vi "10-Tap 8-bit Camera with DRAM (FPGA).vi"() -> ()   [LabVIEW 2013]
doc: "This is the FPGA VI for the 10-Tap 8-Bit Camera with DRAM example. This example demonstrates how to acquire images from a 10-tap, 8-bit, extended configuration, Camera Link camera and transfer the images to the host. This example supports area scan and line scan cameras for both continuous and finite acquisitions.\n\nThis example also demonstrates the use of DRAM as a frame buffer for very high speed acquisitions. Data packing and flow-control are also employed to maximize use of the available DRAM and FIFOs in terms of both memory space and performance.\n\nAdditionally, the example demonstrates the serial server, which allows third-party camera configuration utilities to communicate with the camera using the Camera Link serial interface while this VI is running."
uses:
  <vilib>/rvi/DataTransferAndStorage/Container/XNode/niFpgaContainer.xnode
  <vilib>/Platform/TimedLoop/XDataNode/XDataNode.xnode
  <vilib>/Platform/TimedLoop/XDataNode/timing_clust.ctl
  <vilib>/Platform/TimedLoop/XDataNode/XDNodeRunTimeDep.lvlib
  <vilib>/Platform/TimedLoop/XDataNode/wakeup.ctl
  <vilib>/Platform/TimedLoop/XDataNode/nitl_modes.ctl
  <vilib>/eio/EIONode/EIONode.xnode
  <vilib>/rvi/eio/common/nirviEmuTemplateMethod_errors.vi
  <vilib>/rvi/FIFO/Fifo_Resource/nirvififoEmulationGetNumberOfElementsToRead.vi
  <vilib>/rvi/interface/RandomDataEmulation/nirviRandomDataFpgaReadWriteTemplate.vi
  <vilib>/rvi/FIFO/Fifo_Resource/nirvififoEmulationRead.vi
  <vilib>/rvi/FIFO/Fifo_Resource/nirvififoEmulationWrite.vi
  Common/CL Data to Pixels/10 Tap 8-Bit.vi
  FPGA/10-Tap Data/10-Tap Conversion Enum.ctl
  FPGA/Globals/Accumulated Sector Intensity.vi
  FPGA/Globals/Pixel Location Global.vi
  FPGA/Globals/Sector Parameter Global.vi
  <vilib>/rvi/FIFO/Fifo_Resource/nirvififoEmulationGetNumberOfElementsToWrite.vi
  Common/CL Signal Mapping.ctl
  Common/CL Configuration.ctl
  FPGA/Sector/Accumulate/Sector Parameter Cluster.ctl
panel:
  in  "Right End Angle Duty Cycle":fxp<+,8,0>
  in  "Right Start Angle Duty Cycle":fxp<+,8,0>
  in  "Left End Angle Duty Cycle":fxp<+,8,0>
  in  "Left Start Angle Duty Cycle":fxp<+,8,0>
  in  "X Resolution":u16=1000
  in  "Y Resolution":u16=1000
  out "Analysis Ticks":u32
  out "Right Sector Edge":u8
  out "Left Sector Edge":u8
  in  "[Average BG Intensity]":u8[](array[numeric])=[0, 0, 0, 0, 0, 0, 0, 0, 0, 0, 0, 0, 0, 0, 0, 0, 0, 0, 0, 0, 0, 0, 0, 0, 0, 0, 0, 0, 0, 0, 0, 0]
  in  "Sector Threshold":u8
  in  "# of Frames to Average":u8
  in  "Sector Parameters Right":T1={"Start Angle"=0.0, "End Angle"=0.4708251953125, "Inner Radius"=309, "Outter Radius"=405, "Hinge X"=685, "Hinge Y"=527, "NumWingSectors"=8}
  in  "Sector Parameters Left":T1={"Start Angle"=0.65740966796875, "End Angle"=0.99468994140625, "Inner Radius"=309, "Outter Radius"=405, "Hinge X"=464, "Hinge Y"=534, "NumWingSectors"=8}
  in  "CL Config.Configuration":T2=enum."Full"
  in  "CL Config.Signal Mapping":T3=enum."Basler 10-tap"
  in  "CL Config.Line Scan":bool
  in  "CL Config.DVAL Active High":bool=TRUE
  in  "CL Config.LVAL Active High":bool=TRUE
  in  "CL Config.FVAL Active High":bool=TRUE
  in  "CL Config.Spare Active High":bool=TRUE
  in  "Acq Control.Line Scan Height":u32
  in  "Acq Control.Frames To Acq":u32
  in  "Acq Control.Acquire":bool
  in  "Acq Control.Cancel Acq":bool
  in  "Acq Control.Ignore DVAL":bool
  in  "Acq Control.Initialize":bool
  out "Acq Status.Acq In Progress":bool
  out "Acq Status.Clocks Per Line":u32
  out "Acq Status.Frames Acq'd":u32
  out "Acq Status.Lines Per Frame":u32
  out "Acq Status.DMA Write Timeout":bool
  out "Acq Status.Initialized":bool
  in  "UART.Baud Rate":u8
  in  "UART.Transmit":bool
  in  "UART.Tx Data":u8[](array[numeric])=[0, 0, 0, 0, 0, 0, 0, 0, 0, 0] format="%02x"
  in  "UART.Set Baud Rate":bool
  in  "UART.Byte Mode":bool=TRUE
  out "UART.Rx Ready":bool
  out "UART.Break Indicator":bool
  out "UART.Framing Error":bool
  out "UART.Overrun Error":bool
  out "UART.Tx Ready":bool
  out "UART.Rx Data":u8 format="%02x"
  in  "UART.Receive":bool
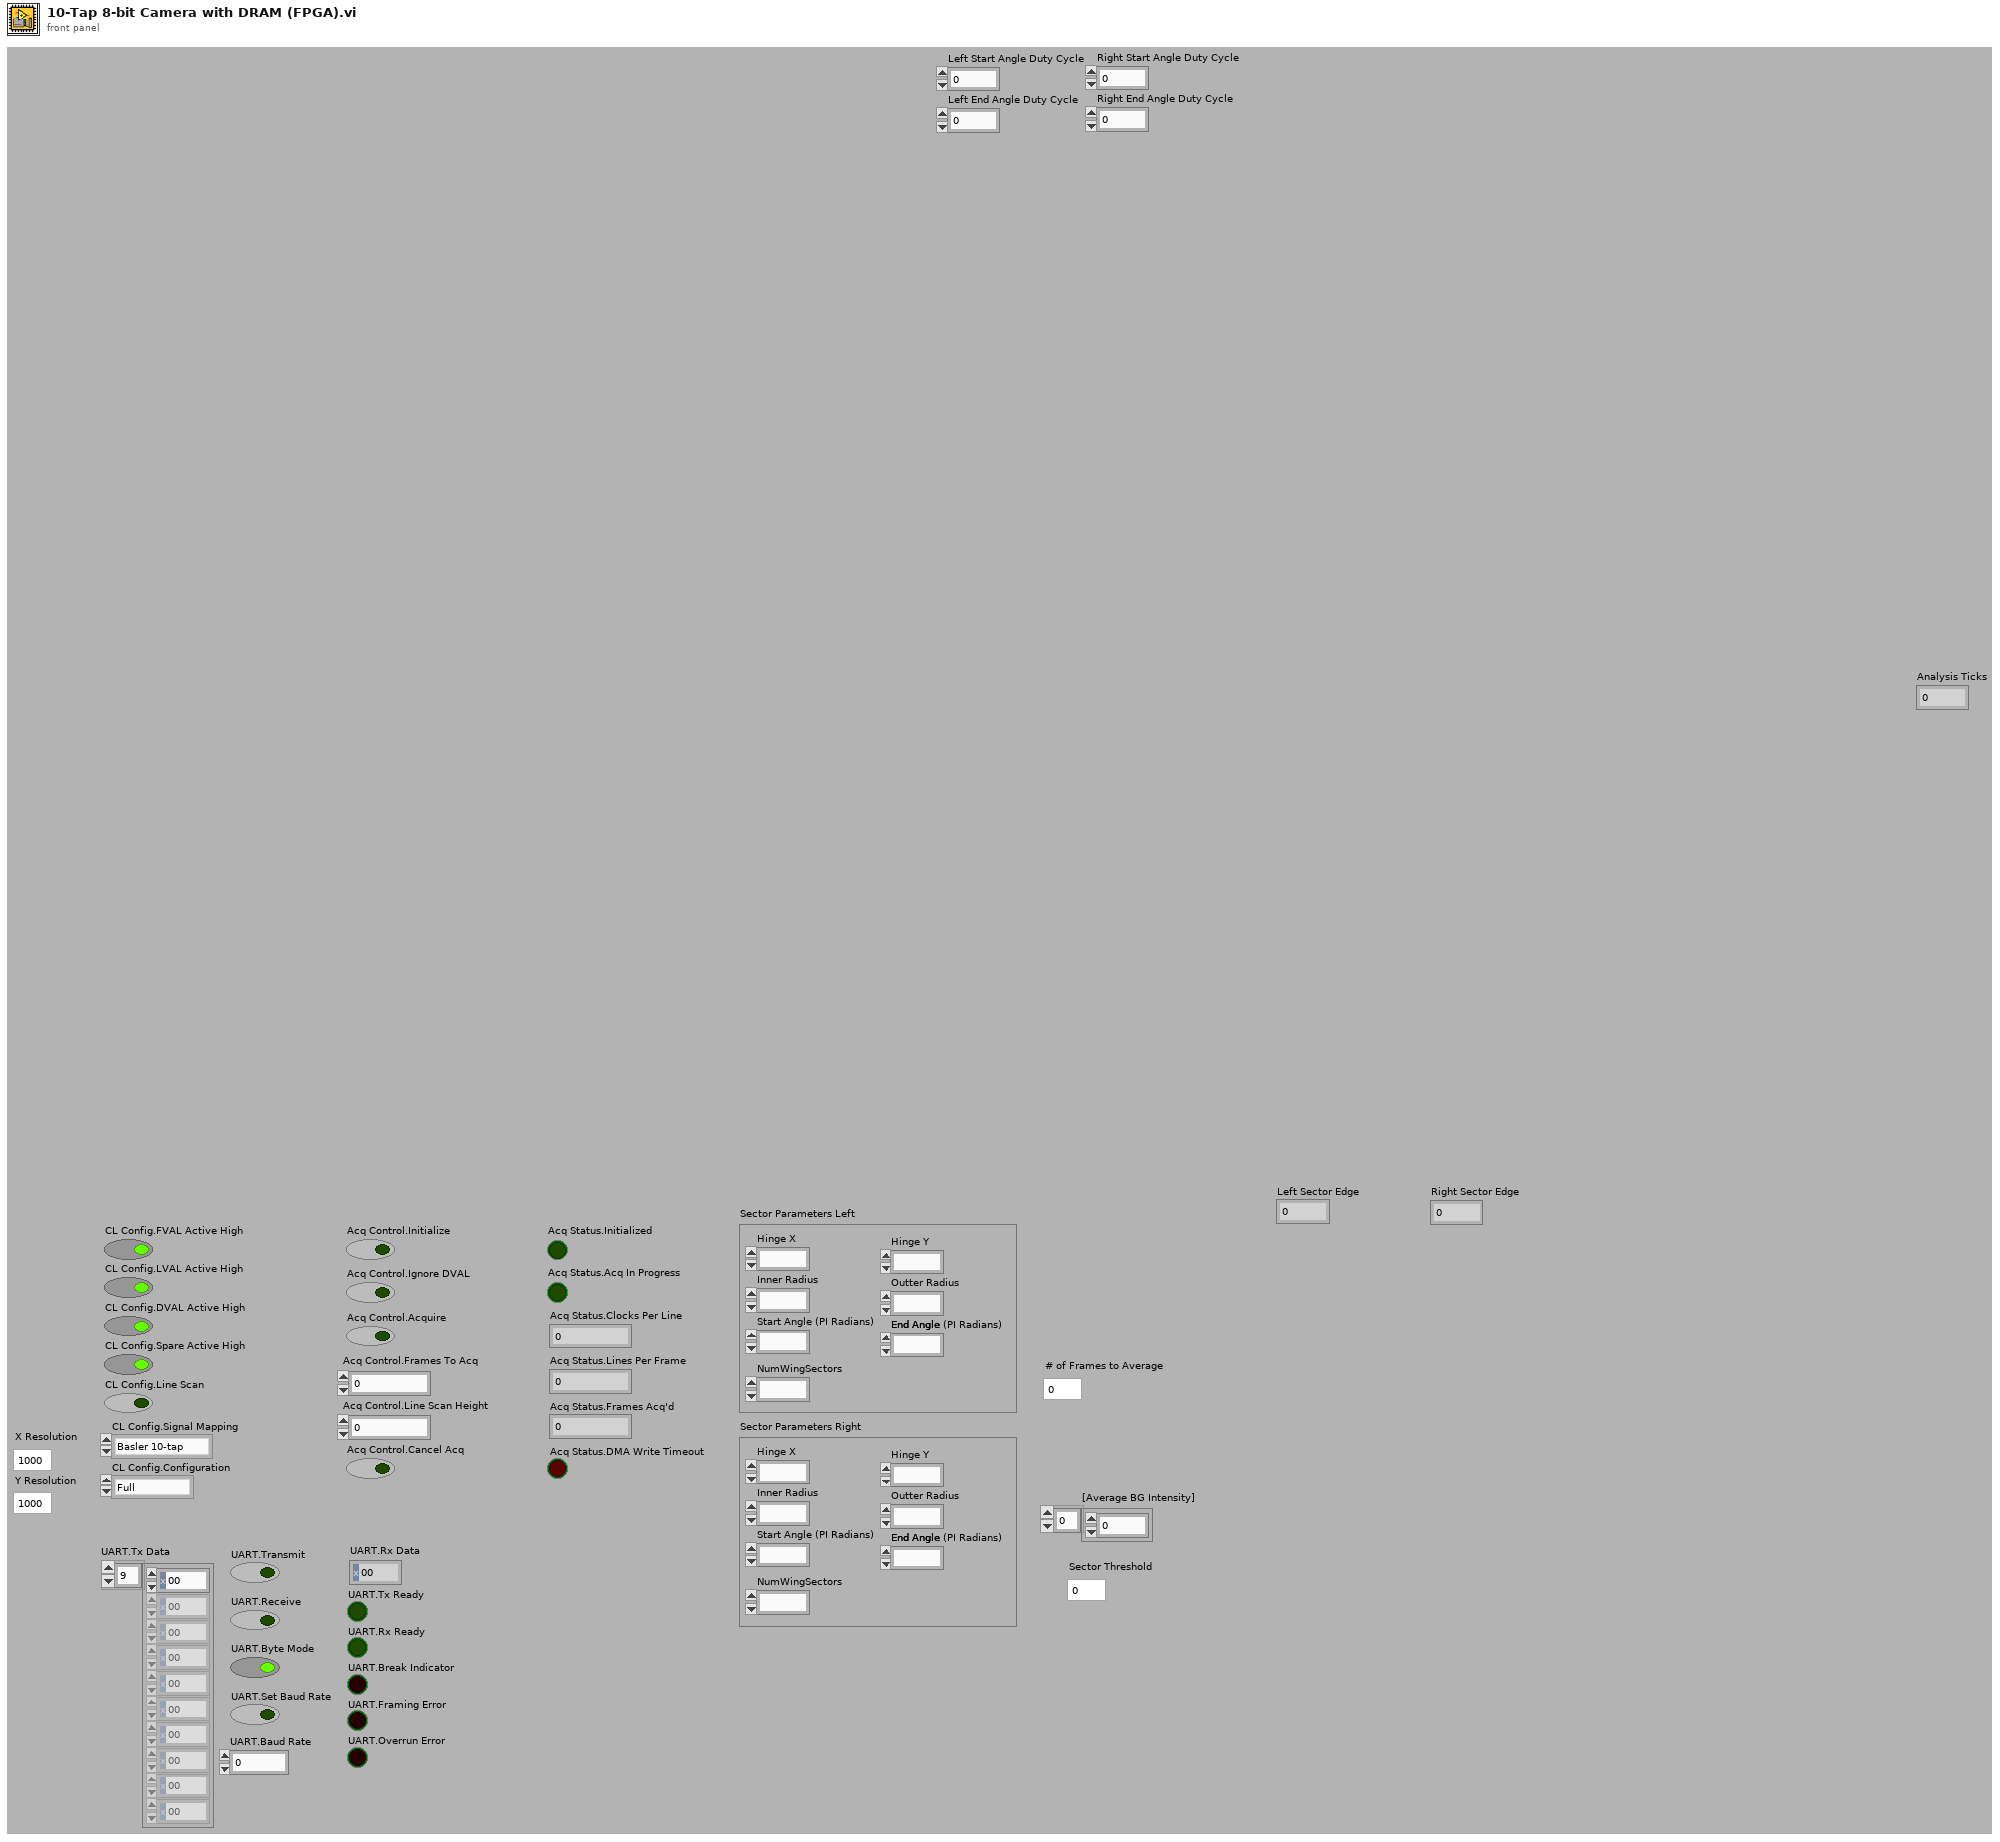
[diagram p1: front panel]
types:
  T1 = typedef "Sector Parameter Cluster.ctl" = cluster{"Start Angle":fxp<+/-,17,2>, "End Angle":fxp<+,17,3>, "Inner Radius":u16, "Outter Radius":u16, "Hinge X":u16, "Hinge Y":u16, "NumWingSectors":u8}
  T2 = typedef "CL Configuration.ctl" = enum8{"Base", "Medium", "Full"}
  T3 = typedef "CL Signal Mapping.ctl" = enum8{"Standard", "Basler 10-tap", "Vosskühler 10-tap"}
  T4 = typedef "XDNodeRunTimeDep.lvlib/timing_clust.ctl" = cluster{"Expected End [f-1]":u64, "Actual End [f-1]":u64, "Finished Late? [f-1]":bool, "Expected End [i-1]":u64, "Actual End [i-1]":u64, "Finished Late? [i-1]":bool, "Expected Start [i]":u64, "Actual Start [i]":u64, "Expected Start [f]":u64, "Actual Start [f]":u64, "Source Name":string, "Structure Name":string, "Period":i64, "Deadline":i64, "Offset":i64, "Start":i64, "Priority":i32, "Timeout":i32, "Mode":T5, "Wakeup Reason":T6, "Error":errorcluster, "Source Type":string, "Secondary Source Type":string, "Global End Time":u64, "Global Start Time":u64, "Frame Duration":u64, "Iteration Duration":u64, "Assigned CPU":i32, "I/O Scan Engine Mode":u32}
  T5 = typedef "XDNodeRunTimeDep.lvlib/nitl_modes.ctl" = enum32{"No Change", "Process missed periods, maintain original phase", "Discard missed periods, maintain original phase", "Process missed periods, ignore original phase", "Discard missed periods, ignore original phase"}
  T6 = typedef "XDNodeRunTimeDep.lvlib/wakeup.ctl" = enum32{"Normal", "Aborted", "Asynchronous wakeup", "Timing source error", "Timed loop error", "Timeout"}
  T7 = typedef "10-Tap Conversion Enum.ctl" = enum16{"10-Tap to 16 and 64", "16 and 64 to 10-Tap"}
  T8 = cluster{"Enables Valid":bool, "Frame Valid":bool, "Line Valid":bool, "Data Valid":bool}
  T9 = typedef "10-Tap 8-bit Cluster.ctl" = cluster{"Pixel 0":u8, "Pixel 1":u8, "Pixel 2":u8, "Pixel 3":u8, "Pixel 4":u8, "Pixel 5":u8, "Pixel 6":u8, "Pixel 7":u8, "Pixel 8":u8, "Pixel 9":u8}
  T10 = cluster{"Tx Data":u8[], "Transmit":bool, "Receive":bool, "Byte Mode":bool, "Set Baud Rate":bool, "Baud Rate":u8}
  T11 = cluster{"Rx Data":u8, "Turn Off Transmit":bool, "Turn Off Receive":bool, "Turn Off Set Baud Rate":bool, "Tx Ready":bool, "Rx Ready":bool, "Break Indicator":bool, "Framing Error":bool, "Overrun Error":bool}
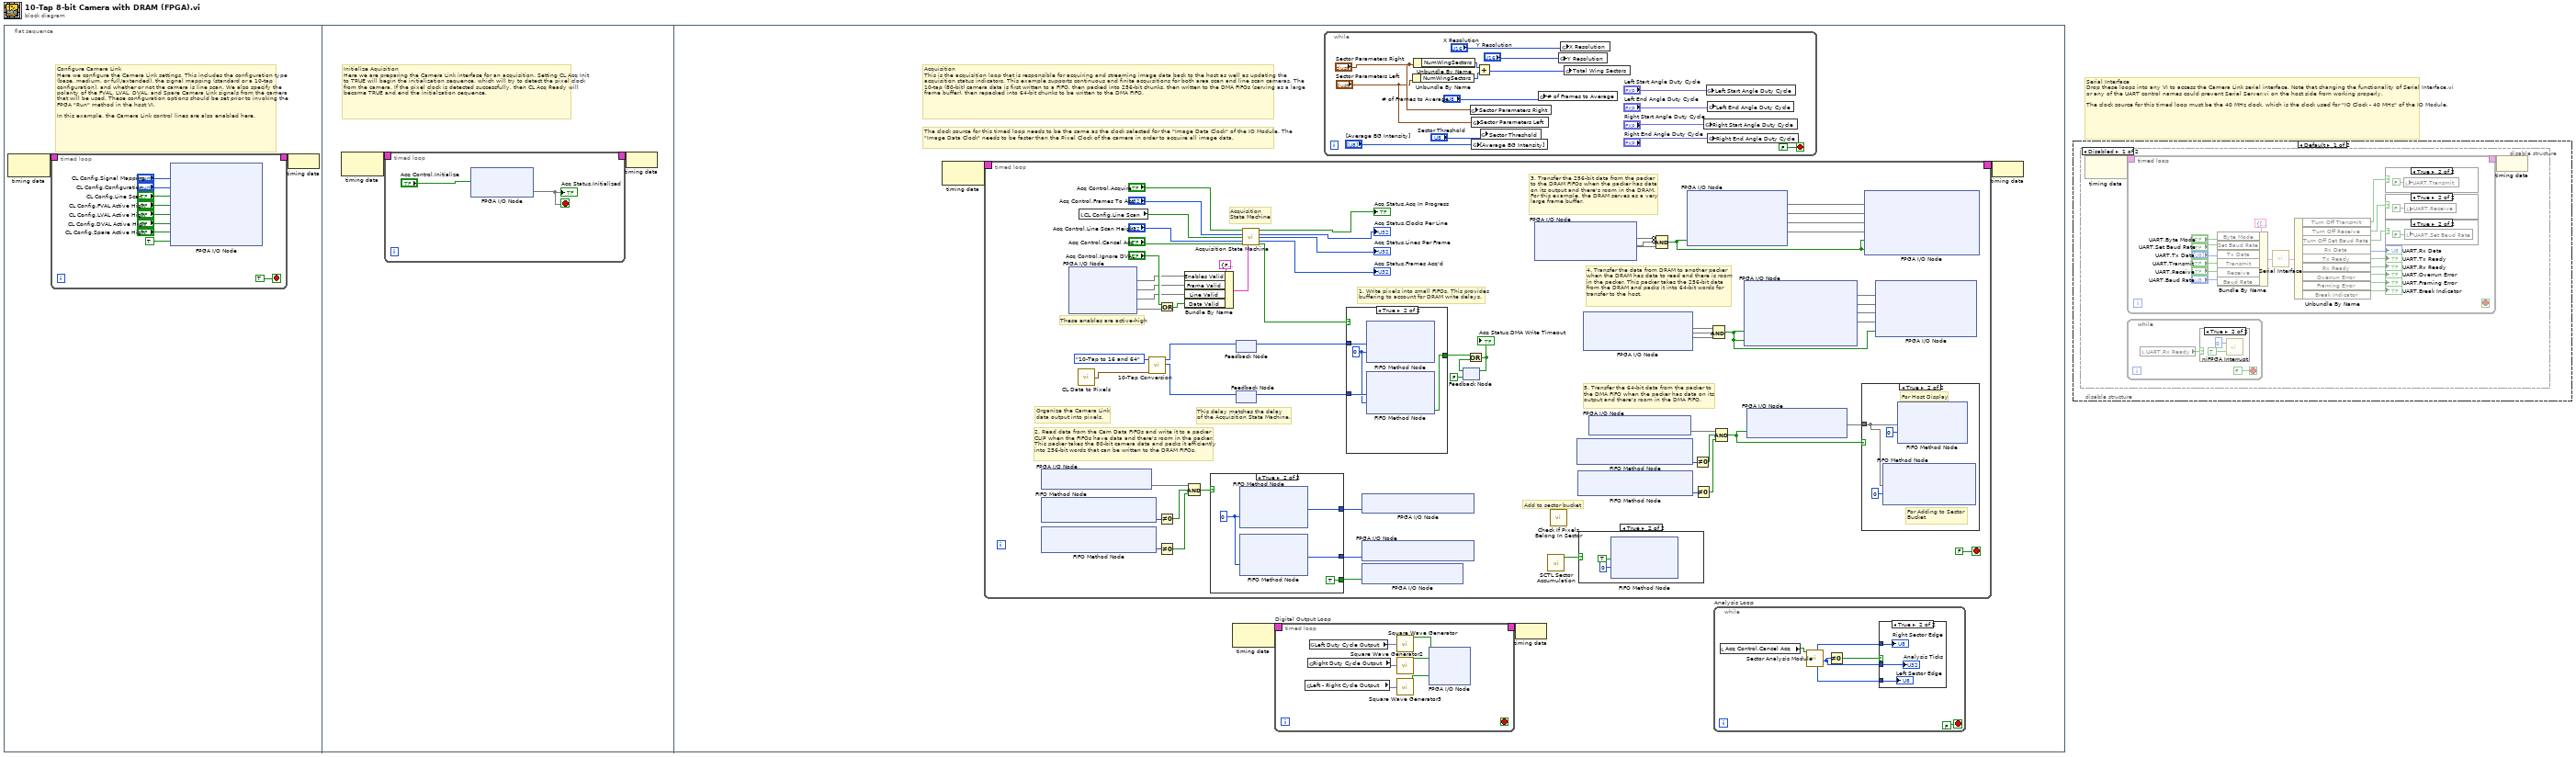
[diagram p0: block diagram]
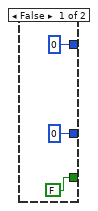
[diagram p11: hidden frame]
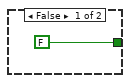
[diagram p12: hidden frame]
diagram:
  # "Serial Interface\nDrop these loops into any VI to access the Camera Link serial interface. Note that changing the functionality of Serial Interface.vi or any of the UART control names could prevent Serial Server.vi on the host side from working properly.\n\nThe clock source for this timed loop must be the 40 MHz clock, which is the clock used for \"IO Clock - 40 MHz\" of the IO Module."
  n1 = flat-sequence {
    frame #0 {
      # "Configure Camera Link\nHere we configure the Camera Link settings. This includes the configuration type (base, medium, or full/extended), the signal mapping (standard or a 10-tap configuration), and whether or not the camera is line scan. We also specify the polarity of the FVAL, LVAL, DVAL, and Spare Camera Link signals from the camera that will be used. These configuration options should be set prior to invoking the FPGA \"Run\" method in the host VI.\n\nIn this example, the Camera Link control lines are also enabled here."
      n2 = node-c288() -> (w2:T4)  [unwired: 1 in]
      n3 = timed-loop {
        timing: w2 -> [_]
        timing-out: [_] -> w1
        stop <- TRUE stop-if-true
        n4 = xnode "FPGA I/O Node"("CL Set Signal Mapping"="CL Config.Signal Mapping", "CL Set Configuration"="CL Config.Configuration", "CL Set Line Scan"="CL Config.Line Scan", "CL Set FVAL Active High"="CL Config.FVAL Active High", "CL Set LVAL Active High"="CL Config.LVAL Active High", "CL Set DVAL Active High"="CL Config.DVAL Active High", "CL Set Spare Active High"="CL Config.Spare Active High", "CL Control Enable"=TRUE ("IO Module\\CL Control Enable")) -> ()  [unwired: 8 in, 8 out]
      }
      n5 = node-c288(w1) -> ()
    }
    frame #1 {
      # "Initialize Aquisition\nHere we are preparing the Camera Link interface for an acquisition. Setting CL Acq Init to TRUE will begin the initialization sequence, which will try to detect the pixel clock from the camera. If the pixel clock is detected successfully, then CL Acq Ready will become TRUE and end the initialzation sequence."
      n6 = node-c288() -> (w17:T4)  [unwired: 1 out]
      n7 = timed-loop {
        timing: w17 -> [_]
        timing-out: [_] -> w16
        stop <- w18 stop-if-true
        n8 = xnode "FPGA I/O Node"("CL Acq Init"="Acq Control.Initialize") -> ("CL Acq Ready"=w18)  [unwired: 2 in, 2 out]
        "Acq Status.Initialized" <- w18
      }
      n9 = node-c288(w16) -> ()
    }
    frame #2 {
      # "The clock source for this timed loop needs to be the same as the clock selected for the \"Image Data Clock\" of the IO Module. The \"Image Data Clock\" needs to be faster than the Pixel Clock of the camera in order to acquire all image data."
      # "Acquisition\nThis is the acquisition loop that is responsible for acquiring and streaming image data back to the host as well as updating the acquisition status indicators. This example supports continuous and finite acquisitions for both area scan and line scan cameras. The 10-tap (80-bit) camera data is first written to a FIFO, then packed into 256-bit chunks, then written to the DMA FIFOs (serving as a large frame buffer), then repacked into 64-bit chunks to be written to the DMA FIFO."
      n10 = node-c288() -> (w27:T4)  [unwired: 1 in]
      n11 = timed-loop {
        timing: w27 -> [_]
        timing-out: [_] -> w26
        stop <- FALSE stop-if-true
        # "These enables are active-high"
        # "Acquisition\nState Machine"
        # "2. Read data from the Cam Data FIFOs and write it to a packer\nCLIP when the FIFOs have data and there's room in the packer.\nThis packer takes the 80-bit camera data and packs it efficiently\ninto 256-bit words that can be written to the DRAM FIFOs."
        # "Organize the Camera Link\ndata output into pixels."
        # "This delay matches the delay\nof the Acquisition State Machine."
        # "Add to sector bucket"
        # "5. Transfer the 64-bit data from the packer to\nthe DMA FIFO when the packer has data on its\noutput and there's room in the DMA FIFO."
        # "4. Transfer the data from DRAM to another packer\nwhen the DRAM has data to read and there is room\nin the packer. This packer takes the 256-bit data\nfrom the DRAM and packs it into 64-bit words for\ntransfer to the host."
        # "3. Transfer the 256-bit data from the packer\nto the DRAM FIFOs when the packer has data\non its output and there's room in the DRAM.\nFor this example, the DRAM serves as a very\nlarge frame buffer."
        # "1. Write pixels into small FIFOs. This provides\nbuffering to account for DRAM write delays."
        n12 = xnode "FPGA I/O Node"() -> ("Pack 80 to 256\\Ready For Write"=w96)  [unwired: 1 in, 1 out]
        n13 = xnode ("FIFO Method Node")() -> ("Number of Elements to Read"=w100:u32)  [unwired: 1 in, 1 out]
        n14 = xnode ("FIFO Method Node")() -> ("Number of Elements to Read"=w99:u32)  [unwired: 1 in, 1 out]
        n15 = xnode "FPGA I/O Node"() -> ("CL Output Valid"=w54, "CL Frame Valid"=w55, "CL Line Valid"=w56, "CL Data Valid"=w59)  [unwired: 4 in, 4 out]
        n16 = call-poly "CL Data to Pixels.vi"() -> ("Pixels"=w47:T9)  [unwired: 1 in]
        n17 = local read "CL Config.Line Scan"() -> (w62:bool)
        n18 = call "10-Tap Conversion.vi"("10 Tap In"=w47, "Operation"=10-Tap_Conversion_Enum."10-Tap to 16 and 64") -> ("64 Bit Out"=w48:u64, "16 Bit Out"=w49:u16)  [unwired: 7 in, 1 out]
        n19 = Or(x="Acq Control.Ignore DVAL", y=w59) -> (x .or. y?=w60:bool)
        n20 = Not Equal To 0?(x=w100) -> (x != 0?=w94:bool)
        n21 = Not Equal To 0?(x=w99) -> (x != 0?=w93:bool)
        n22 = Bundle By Name(cluster=T8 {"Enables Valid"=FALSE, "Frame Valid"=FALSE, "Line Valid"=FALSE, "Data Valid"=FALSE} ("Enables"), "Enables Valid"=w54, "Frame Valid"=w55, "Line Valid"=w56, "Data Valid"=w60) -> (w57:T8)
        n23 = Compound Arithmetic op=AND(w96, w94, w93) -> (w95:bool)
        n24 = case shown="True" w95 {
          tunnel: [u16 0 ("Element") w119] -> w101
          tunnel: [u64 0 ("Element") w118] -> w97
          tunnel: [FALSE TRUE] -> w98
          frame False {
          }
          frame True {
            w117 = 0 ("Timeout")
            n25 = xnode ("FIFO Method Node")("Timeout"=w117) -> ("Element"=w119:u16)  [unwired: 1 in, 2 out]
            n26 = xnode ("FIFO Method Node")("Timeout"=w117) -> ("Element"=w118:u64)  [unwired: 1 in, 2 out]
          }
        }
        n27 = feedback #1() -> (w102:u16)  [unwired: 1 in]
        n28 = feedback-in #1(w49) -> ()
        n29 = feedback #2() -> (w107:u64)  [unwired: 1 in]
        n30 = feedback-in #2(w48) -> ()
        n31 = call "Acquisition State Machine.vi"("Acquire"="Acq Control.Acquire", "Frames to Acquire"="Acq Control.Frames To Acq", "Line Scan"=w62, "Line Scan Height"="Acq Control.Line Scan Height", "Cancel Acq"="Acq Control.Cancel Acq", "Enables"=w57) -> ("Acq In Progress"=→"Acq Status.Acq In Progress":bool, "Num Clocks Per Line"=→"Acq Status.Clocks Per Line":u32, "Num Lines Per Frame"=→"Acq Status.Lines Per Frame":u32, "Num Frames Acq'd"=→"Acq Status.Frames Acq'd":u32, "Capture Cycle"=w91:bool)  [unwired: 4 in, 1 out]
        n32 = case shown="True" w91 {
          tunnel: [FALSE ("Timed Out?") w123] -> w105
          tunnel: w107 -> [_ w124]
          tunnel: w102 -> [_ w122]
          frame False {
          }
          frame True {
            w121 = 0 ("Timeout")
            n33 = xnode ("FIFO Method Node")("Element"=w122, "Timeout"=w121) -> ()  [unwired: 1 in, 2 out]
            n34 = xnode ("FIFO Method Node")("Element"=w124, "Timeout"=w121) -> ("Timed Out?"=w123:bool)  [unwired: 1 in, 1 out]
          }
        }
        n35 = xnode "FPGA I/O Node"("Pack 80 to 256\\Data In Upper 16"=w101) -> ()  [unwired: 1 in, 1 out]
        n36 = xnode "FPGA I/O Node"("Pack 80 to 256\\Data In Lower 64"=w97) -> ()  [unwired: 1 in, 1 out]
        n37 = xnode "FPGA I/O Node"("Pack 80 to 256\\Write Enable"=w98) -> ()  [unwired: 1 in, 1 out]
        n38 = feedback #3(FALSE) -> (w104:bool)
        n39 = Or(x=w105, y=w104) -> (x .or. y?=w103:bool)
        "Acq Status.DMA Write Timeout" <- w103
        n40 = feedback-in #3(w103) -> ()
        n41 = xnode "FPGA I/O Node"() -> ("DRAM Bank 0\\Full"=w67, "Pack 80 to 256\\Output Valid"=w86)  [unwired: 3 in, 4 out]
        n42 = call "SCTL Sector Accumulation.vi"() -> ("New Data?"=w64:bool)  [unwired: 11 in]
        n43 = call "Check If Pixels Belong In Sector.vi"() -> ()  [unwired: 11 in, 1 out]
        n44 = xnode ("FIFO Method Node")() -> ("Number of Elements to Write"=w69:u32)  [unwired: 1 in, 1 out]
        n45 = xnode ("FIFO Method Node")() -> ("Number of Elements to Write"=w66:u32)  [unwired: 1 in, 1 out]
        n46 = case shown="True" w64 {
          frame False {
          }
          frame True {
            n47 = xnode ("FIFO Method Node")("Element"=TRUE, "Timeout"=0) -> ()  [unwired: 1 in, 2 out]
          }
        }
        n48 = xnode "FPGA I/O Node"() -> ("DRAM Bank 1\\Data_Available"=w80, "DRAM Bank 0\\Data_Available"=w78, "Pack 256 to 64\\Ready for Write"=w79)  [unwired: 3 in, 3 out]
        n49 = xnode "FPGA I/O Node"() -> ("Pack 256 to 64\\Output Valid"=w71)  [unwired: 1 in, 1 out]
        n50 = Compound Arithmetic op=AND(invert w67, invert w67, w86) -> (w81:bool)
        n51 = xnode "FPGA I/O Node"("Pack 80 to 256\\Read Enable"=w81) -> ("Pack 80 to 256\\Data Out 3"=w85, "Pack 80 to 256\\Data Out 2"=w84, "Pack 80 to 256\\Data Out 1"=w83, "Pack 80 to 256\\Data Out 0"=w82)  [unwired: 5 in, 5 out]
        n52 = Not Equal To 0?(x=w69) -> (x != 0?=w70:bool)
        n53 = Not Equal To 0?(x=w66) -> (x != 0?=w65:bool)
        n54 = Compound Arithmetic op=AND(w80, w78, w79) -> (w73:bool)
        n55 = Compound Arithmetic op=AND(w71, w70, w65) -> (w68:bool)
        n56 = xnode "FPGA I/O Node"("DRAM Bank 1\\Read"=w73, "DRAM Bank 0\\Read"=w73) -> ("DRAM Bank 1\\Read_Data_Upper"=w77, "DRAM Bank 1\\Read_Data_Lower"=w76, "DRAM Bank 0\\Read_Data_Upper"=w75, "DRAM Bank 0\\Read_Data_Lower"=w74)  [unwired: 6 in, 6 out]
        n57 = xnode "FPGA I/O Node"("Pack 256 to 64\\Read Enable"=w68) -> ("Pack 256 to 64\\Data Out 64"=w72)  [unwired: 2 in, 2 out]
        n58 = case shown="True" w68 {
          tunnel: w72 -> [_ w111]
          frame False {
          }
          frame True {
            # "For Adding to Sector \nBucket"
            # "For Host Display"
            n59 = xnode ("FIFO Method Node")("Element"=w111, "Timeout"=0) -> ()  [unwired: 1 in, 2 out]
            n60 = xnode ("FIFO Method Node")("Element"=w111, "Timeout"=0) -> ()  [unwired: 1 in, 2 out]
          }
        }
        n61 = xnode "FPGA I/O Node"("DRAM Bank 1\\Write_Data_Upper"=w85, "DRAM Bank 1\\Write_Data_Lower"=w84, "DRAM Bank 0\\Write_Data_Upper"=w83, "DRAM Bank 0\\Write_Data_Lower"=w82, "DRAM Bank 1\\Write"=w81, "DRAM Bank 0\\Write"=w81) -> ()  [unwired: 6 in, 6 out]
        n62 = xnode "FPGA I/O Node"("Pack 256 to 64\\Data In 3"=w77, "Pack 256 to 64\\Data In 2"=w76, "Pack 256 to 64\\Data In 1"=w75, "Pack 256 to 64\\Data In 0"=w74, "Pack 256 to 64\\Write Enable"=w73) -> ()  [unwired: 5 in, 5 out]
      }
      n63 = node-c288() -> (w25:T4)  [unwired: 1 in]
      n64 = timed-loop "Digital Output Loop" {
        timing: w25 -> [_]
        timing-out: [_] -> w24
        stop <- _ stop-if-true
        n65 = global read "Sector Parameter Global.vi" "Left - Right Cycle Output"() -> (w40:fxp<+,8,0>)
        n66 = global read "Sector Parameter Global.vi" "Right Duty Cycle Output"() -> (w41:fxp<+,8,0>)
        n67 = global read "Sector Parameter Global.vi" "Left Duty Cycle Output"() -> (w42:fxp<+,8,0>)
        n68 = call "Square Wave Generator"("duty cycle (periods)"=w42) -> ("square wave out"=w39:bool)  [unwired: 14 in]
        n69 = call "Square Wave Generator2"("duty cycle (periods)"=w41) -> ("square wave out"=w38:bool)  [unwired: 14 in]
        n70 = call "Square Wave Generator3"("duty cycle (periods)"=w40) -> ("square wave out"=w37:bool)  [unwired: 14 in]
        n71 = xnode "FPGA I/O Node"("TTL 0"=w39, "TTL 1"=w38, "TTL 2"=w37) -> ()  [unwired: 3 in, 3 out]
      }
      n72 = while {
        stop <- FALSE stop-if-true
        n73 = Unbundle By Name("Sector Parameters Left") -> ("NumWingSectors"=w141:u8)
        n74 = Unbundle By Name("Sector Parameters Right") -> ("NumWingSectors"=w142:u8)
        n75 = global write "Sector Parameter Global.vi" "Sector Parameters Right"("Sector Parameters Right") -> ()
        n76 = global write "Sector Parameter Global.vi" "Sector Parameters Left"("Sector Parameters Left") -> ()
        n77 = global write "Sector Parameter Global.vi" "[Average BG Intensity]"("[Average BG Intensity]") -> ()
        n78 = Add(x=w142, y=w141) -> (x+y=w140:u8)
        n79 = global write "Sector Parameter Global.vi" "Sector Threshold"("Sector Threshold") -> ()
        n80 = global write "Pixel Location Global.vi" "# of Frames to Average"("# of Frames to Average") -> ()
        n81 = global write "Pixel Location Global.vi" "Y Resolution"("Y Resolution") -> ()
        n82 = global write "Pixel Location Global.vi" "X Resolution"("X Resolution") -> ()
        n83 = global write "Accumulated Sector Intensity.vi" "Total Wing Sectors"(w140) -> ()
        n84 = global write "Sector Parameter Global.vi" "Right Start Angle Duty Cycle"("Right Start Angle Duty Cycle") -> ()
        n85 = global write "Sector Parameter Global.vi" "Left Start Angle Duty Cycle"("Left Start Angle Duty Cycle") -> ()
        n86 = global write "Sector Parameter Global.vi" "Left End Angle Duty Cycle"("Left End Angle Duty Cycle") -> ()
        n87 = global write "Sector Parameter Global.vi" "Right End Angle Duty Cycle"("Right End Angle Duty Cycle") -> ()
      }
      n88 = node-c288(w24) -> ()
      n89 = while "Analysis Loop" {
        stop <- FALSE stop-if-true
        n90 = local read "Acq Control.Cancel Acq"() -> (w32:bool)
        n91 = call "Sector Analysis Module.vi"("Canceled?"=w32) -> ("Analysis Ticks"=w31:u32, "Left Sector Edge"=w28:u8, "Right Sector Edge"=w29:u8)  [unwired: 6 in, 2 out]
        n92 = Not Equal To 0?(x=w31) -> (x != 0?=w30:bool)
        n93 = case shown="True" w30 {
          tunnel: w31 -> [_ w36]
          tunnel: w29 -> [_ w35]
          tunnel: w28 -> [_ w34]
          frame False {
          }
          frame True {
            "Analysis Ticks" <- w36
            "Right Sector Edge" <- w35
            "Left Sector Edge" <- w34
          }
        }
      }
      n94 = node-c288(w26) -> ()
    }
  }
  n95 = disable-structure shown="Default" {
    frame condition #0 {
      n96 = disable-structure shown="Disabled" {
        frame Disabled {
          n97 = node-c288() -> (w145:T4)  [unwired: 1 out]
          n98 = timed-loop {
            timing: w145 -> [_]
            timing-out: [_] -> w144
            stop <- _ stop-if-true
            n99 = Bundle By Name(cluster=T10 {"Tx Data"=[0, 0, 0, 0, 0, 0, 0, 0, 0, 0], "Transmit"=FALSE, "Receive"=FALSE, "Byte Mode"=TRUE, "Set Baud Rate"=FALSE, "Baud Rate"=0} ("UART Inputs"), "Byte Mode"="UART.Byte Mode", "Set Baud Rate"="UART.Set Baud Rate", "Tx Data"="UART.Tx Data", "Transmit"="UART.Transmit", "Receive"="UART.Receive", "Baud Rate"="UART.Baud Rate") -> (w150:T10)
            n100 = call "Serial Interface.vi"("UART Inputs"=w150) -> ("UART Outputs"=w162:T11)
            n101 = Unbundle By Name(w162) -> ("Turn Off Transmit"=w155:bool, "Turn Off Receive"=w156:bool, "Turn Off Set Baud Rate"=w152:bool, "Rx Data"=→"UART.Rx Data":u8, "Tx Ready"=→"UART.Tx Ready":bool, "Rx Ready"=→"UART.Rx Ready":bool, "Overrun Error"=→"UART.Overrun Error":bool, "Framing Error"=→"UART.Framing Error":bool, "Break Indicator"=→"UART.Break Indicator":bool)
            n102 = case shown="True" w155 {
              frame False {
              }
              frame True {
                n103 = local write "UART.Transmit"(FALSE ("UART.Transmit")) -> ()
              }
            }
            n104 = case shown="True" w156 {
              frame False {
              }
              frame True {
                n105 = local write "UART.Receive"(FALSE ("UART.Receive")) -> ()
              }
            }
            n106 = case shown="True" w152 {
              frame False {
              }
              frame True {
                n107 = local write "UART.Set Baud Rate"(FALSE ("UART.Receive")) -> ()
              }
            }
          }
          n108 = while {
            stop <- FALSE stop-if-true
            n109 = local read "UART.Rx Ready"() -> (w147:bool)
            n110 = case shown="True" w147 {
              frame False {
              }
              frame True {
                n111 = call <vilib>:"niFPGA Interrupt.vi"("Wait Until Cleared (F)"=TRUE ("Wait Until Cleared"), "IRQ Number (0)"=u8 0 ("IRQ Number")) -> ()  [unwired: 1 in]
              }
            }
          }
          n112 = node-c288(w144) -> ()
        }
        frame Enabled {
        }
      }
    }
    frame condition #1 (active) {
    }
  }
